vi "Update Root Message.vi"(8 "error in (no error)":errorcluster, 10 "Message":string, 11 "Root in":refnum<class "Root.lvclass">) -> (0 "error out":errorcluster, 3 "Root out":refnum<class "Root.lvclass">)   [LabVIEW 2025, in "Root.lvlib" / "Root.lvclass"]
uses:
  Root.lvclass
  Root.lvclass/Root.ctl
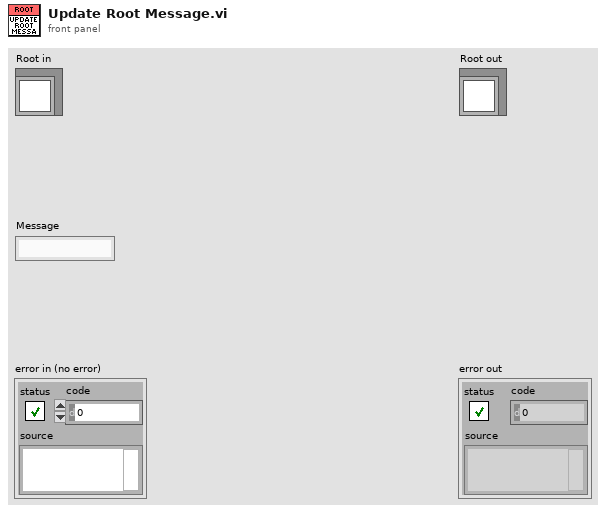
[diagram p1: front panel]
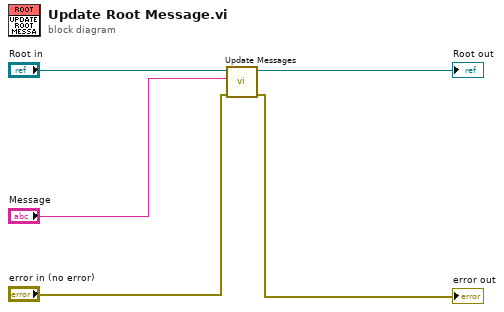
[diagram p0: block diagram]
diagram:
  n1 = call-dynamic "Update Messages.vi"("error in (no error)"="error in (no error)", "Message"="Message", "Root in"="Root in") -> ("error out"=→"error out":errorcluster, "Root out"=→"Root out":refnum<class "Root.lvclass">)  [unwired: 7 in]
